vi "ResetDeadlockBlocker.vi"(8 "error in (no error)":errorcluster, 10 "MaxDeadloopValue":i32=10, 11 "BME_DG_System in":refnum<class "BME_DG_System.lvclass">) -> (0 "error out":errorcluster, 3 "BME_DG_System out":refnum<class "BME_DG_System.lvclass">)   [LabVIEW 2009, in "POLARIS BME DG.lvlib" / "BME_DG_System.lvclass"]
doc: "The VI resets DeadloopBlocker and set MaxDeadloopValue.\n\nCall this VI before You performe delay dependencies check.\n\n----------------------------\n\nauthor: Alexander Kessler, Helmholtz-Institut-Jena \nmaintainer: Alexander Kessler: alexander.kessler@uni-jena.de\n\nLast Change:\nLicense Agreement for this software:\n\nCopyright (C)\nHelmholtz-Institut-Jena\nFröbelsteg 3\n07743 Jena\nGermany\n\nContact: alexander.kessler@uni-jena.de\n\nThis program is free software; you can redistribute it and/or modify it under the terms of the GNU General Public License as published by the Free Software Foundation; either version 2 of the license, or (at your option) any later version.\n\nThis program is distributed in the hope that it will be useful, but WITHOUT ANY WARRANTY; without even the implied warranty of MERCHANTABILITY or FITNESS FOR A PARTICULAR PURPOSE. See the GNU General License for more details (http://www.gnu.org)."
uses:
  BME_DG_System.lvclass
  BME_DG_System.lvclass/BME_DG_System.ctl
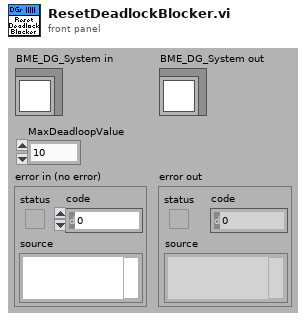
[diagram p1: front panel]
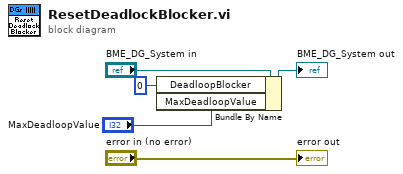
[diagram p0: block diagram]
diagram:
  n1 = Bundle By Name(cluster="BME_DG_System in", "DeadloopBlocker"=0, "MaxDeadloopValue"="MaxDeadloopValue") -> (→"BME_DG_System out":refnum<class "BME_DG_System.lvclass">)
  "error out" <- "error in (no error)"
